vi "Untitled 1.vi"() -> ()   [LabVIEW 2016]
uses:
  controls/data control cluster.ctl
panel:
  out "sequence result header":string[](array[string])
  out "sequence  Result":dbl[][](array[numeric])
  out "DATA CLUSTER out":T1
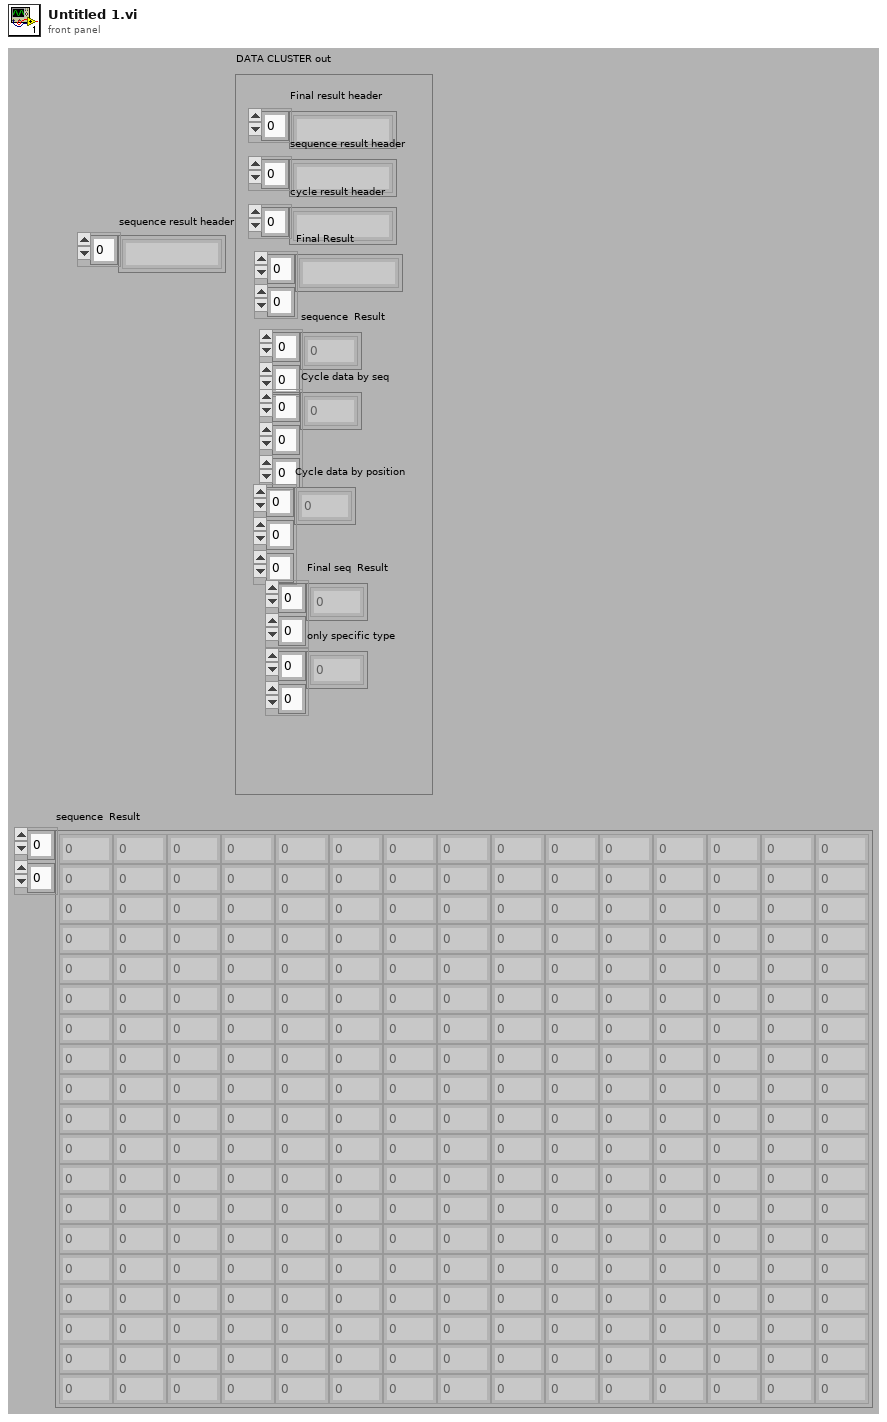
[diagram p1: front panel]
types:
  T1 = typedef "data control cluster.ctl" = cluster{"Final result header":string[], "sequence result header":string[], "cycle result header ":string[], "Final Result":string[][], "sequence  Result":dbl[][], "Cycle data by seq":dbl[][][], "Cycle data by position":dbl[][][], "Final seq  Result":dbl[][], "only specific type":dbl[][]}
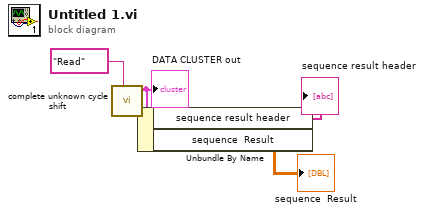
[diagram p0: block diagram]
diagram:
  n1 = call "complete unknown cycle shift.vi"("read write shift"="Read") -> ("DATA CLUSTER out"=w3:T1)  [unwired: 9 in, 1 out]
  "DATA CLUSTER out" <- w3
  n2 = Unbundle By Name(w3) -> ("sequence result header"=→"sequence result header":string[], "sequence  Result"=→"sequence  Result":dbl[][])
